vi "goalExists.vi"(8 "error in (no error)":errorcluster, 10 "Goal.lvclass":refnum<class "Goal.lvclass">, 11 "Account History in":refnum<class "Account History.lvclass">) -> (0 "error out":errorcluster, 2 "Exists?":bool, 3 "Account History out":refnum<class "Account History.lvclass">)   [LabVIEW 2020, in "Account History.lvclass"]
uses:
  Account History.lvclass
  Goal/Goal.lvclass
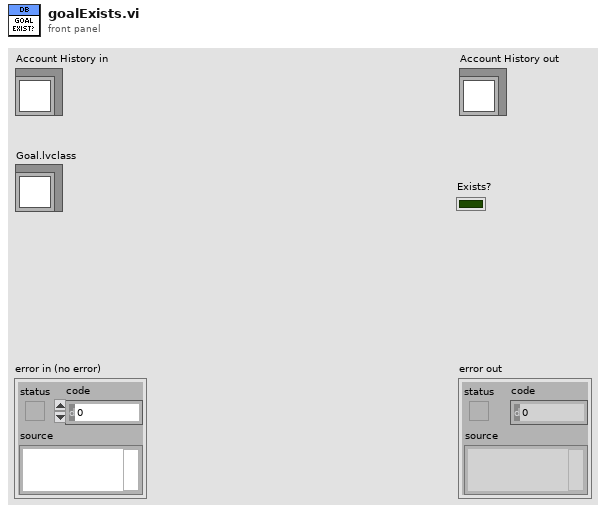
[diagram p1: front panel]
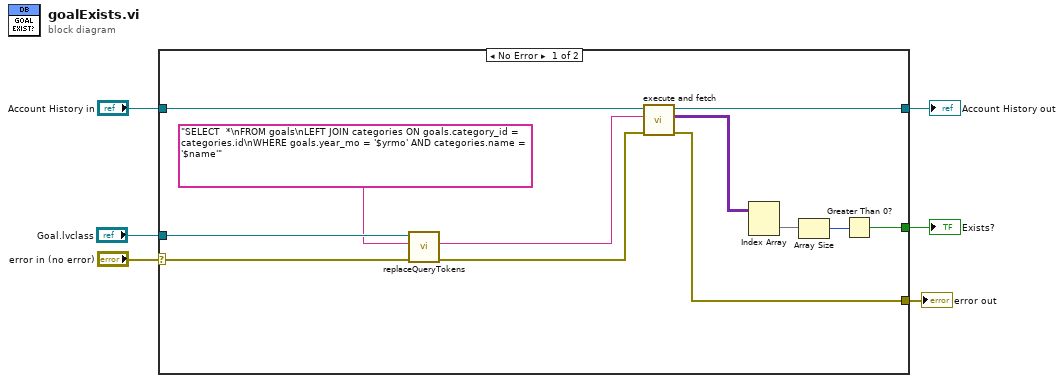
[diagram p0: block diagram]
diagram:
  n1 = case shown="No Error" "error in (no error)" {
    selector: "error in (no error)" -> [w9 w20]
    tunnel: [w16 w20] -> w5
    tunnel: [w17 w19] -> w3
    tunnel: "Account History in" -> [w18 w19]
    tunnel: [w12 _] -> w2
    tunnel: "Goal.lvclass" -> [w11 _]
    frame No Error {
      n2 = call "replaceQueryTokens.vi"("error in (no error)"=w9, "Querry In"="SELECT  *\nFROM goals\nLEFT JOIN categories ON goals.category_id = categories.id\nWHERE goals.year_mo = '$yrmo' AND categories.name = '$name'", "Goal in"=w11) -> ("error out"=w7:errorcluster, "Query Out"=w8:string)  [unwired: 6 in, 1 out]
      n3 = call "execute and fetch.vi"("error in (no error)"=w7, "SQL query"=w8, "Database in"=w18) -> ("error out"=w16:errorcluster, "recordset data"=w15:variant[][], "Database out"=w17:refnum<class "Account History.lvclass">)  [unwired: 6 in]
      n4 = Index Array(array=w15) -> (element=w14:variant[])  [unwired: 2 in]
      n5 = Array Size(array=w14) -> (size(s)=w13:i32)
      n6 = Greater Than 0?(x=w13) -> (x > 0?=w12:bool)
    }
    frame Error {
    }
  }
  "error out" <- w5
  "Account History out" <- w3
  "Exists?" <- w2
